vi "PalmSense Configure EIS.vi"(8 "error in (no error)":errorcluster, 10 "Message Data":variant, 11 "Data Cluster in":T1) -> (0 "error out":errorcluster, 3 "Data Cluster out":T1)   [LabVIEW 2020, in "PalmSens.lvlib"]
uses:
  PalmSens.lvlib
  PalmSense Hardware Configuration.ctl
  <instrlib>/PalmSens SDK for LabVIEW 5.10/PalmSens/PalmSens.lvclass
  support/Message Queue/Message Cluster.ctl
  support/HW Message Cluster.ctl
  C:/Program Files (x86)/National Instruments/LabVIEW 2020/instr.lib/PalmSens SDK for LabVIEW 5.10/PalmSens/Libraries/PalmSens.Core.dll
  support/Message Queue/Message Queue.lvlib
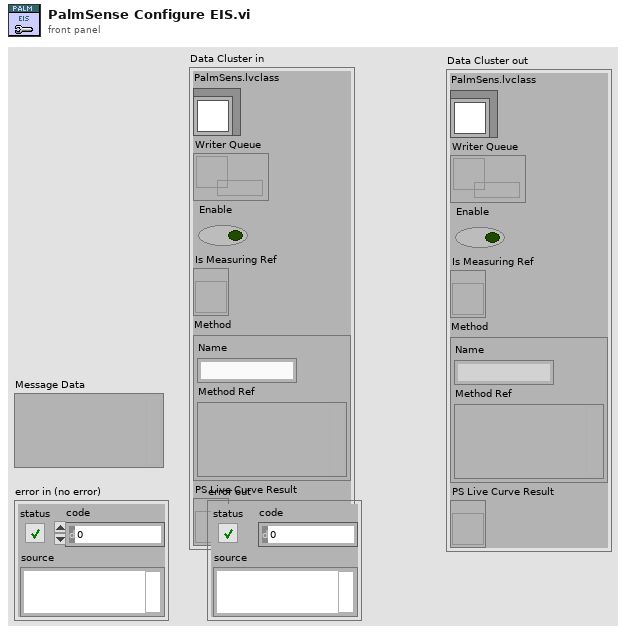
[diagram p1: front panel]
types:
  T1 = typedef "PalmSens.lvlib/PalmSense Hardware Configuration.ctl" = cluster{"PalmSens.lvclass":refnum<class "PalmSens.lvclass">, "Writer Queue":refnum<queue>, "Enable":bool, "Is Measuring Ref":refnum<vi>, "Method":cluster{"Name":string, "Method Ref":variant}, "PS Live Curve Result":refnum<vi>}
  T2 = typedef "Message Queue.lvlib/HW Message Cluster.ctl" = cluster{"Writer Queue":refnum<queue>, "Writer Data":T3}
  T3 = typedef "Message Queue.lvlib/Message Cluster.ctl" = cluster{"Message":string, "Message Data":variant}
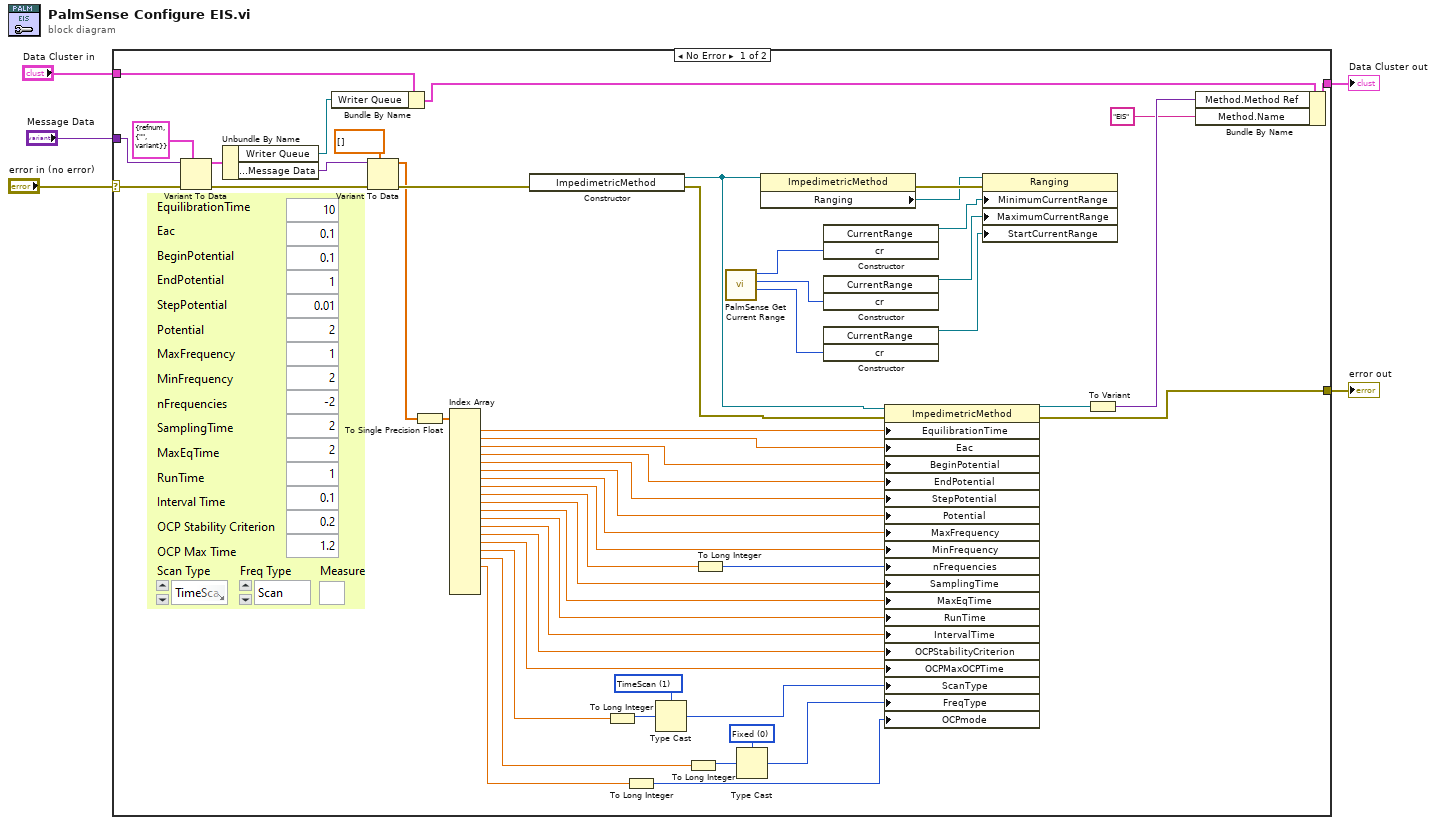
[diagram p0: block diagram]
diagram:
  n1 = case shown="No Error" "error in (no error)" {
    selector: "error in (no error)" -> [w56 w60]
    tunnel: "Message Data" -> [w54 _]
    tunnel: [w42 w61] -> w4
    tunnel: "Data Cluster in" -> [w58 w61]
    tunnel: [w45 w60] -> w2
    frame No Error {
      w32 = 0 items=["Fixed", "Scan"] ("FreqType")
      w34 = 1 items=["PGScan", "TimeScan", "Fixed"] ("ScanType")
      n2 = Variant To Data(error in=w56, type=T2 {"Writer Queue"=refnum, "Writer Data"={"Message"="", "Message Data"=variant}}, Variant=w54) -> (data=w57:T2, error out=w55:errorcluster)
      n3 = Unbundle By Name(w57) -> ("Writer Queue"=w52:refnum<queue>, "Writer Data.Message Data"=w53:variant)
      n4 = Bundle By Name(cluster=w58, "Writer Queue"=w52) -> (w59:T1)
      n5 = Variant To Data(error in=w55, type=dbl[] [] ("LSV Scan"), Variant=w53) -> (data=w37:dbl[], error out=w50:errorcluster)
      n6 = To Single Precision Float(number=w37) -> (single precision float=w27:sgl[])
      n7 = Index Array(array=w27) -> (element #1=w28:sgl, element #2=w26:sgl, element #3=w25:sgl, element #4=w24:sgl, element #5=w23:sgl, element #6=w22:sgl, element #7=w21:sgl, element #8=w20:sgl, element #9=w19:sgl, element #10=w17:sgl, element #11=w16:sgl, element #12=w15:sgl, element #13=w14:sgl, element #14=w13:sgl, element #15=w12:sgl, element #16=w10:sgl, element #17=w8:sgl, element #18=w7:sgl)  [unwired: 21 in, 3 out]
      n8 = constructor class="ImpedimetricMethod"(error in=w50) -> (reference out=w48:refnum<k24>, error out=w49:errorcluster)  [unwired: 2 in, 1 out]
      n9 = To Long Integer(number=w10) -> (32bit integer=w35:i32)
      n10 = To Long Integer(number=w7) -> (32bit integer=w6:i32)
      n11 = Type Cast(type=w34, x=w35) -> (*(type *) &x=w11:i32)
      n12 = To Long Integer(number=w8) -> (32bit integer=w33:i32)
      n13 = To Long Integer(number=w19) -> (32bit integer=w18:i32)
      n14 = call "PalmSense Get Current Range.vi"() -> ("Start Current Range"=w29:i32, "Max Current Range"=w30:i32, "Min Current Range"=w31:i32)  [unwired: 9 in]
      n15 = Type Cast(type=w32, x=w33) -> (*(type *) &x=w9:i32)
      n16 = property class="ImpedimetricMethod"(reference=w48) -> (error out=w47:errorcluster, "Ranging"=w46:refnum<k24>)  [unwired: 1 in, 1 out]
      n17 = constructor class="CurrentRange"("cr"=w31) -> (reference out=w36:refnum<k24>)  [unwired: 3 in, 3 out]
      n18 = constructor class="CurrentRange"("cr"=w30) -> (reference out=w44:refnum<k24>)  [unwired: 3 in, 3 out]
      n19 = constructor class="CurrentRange"("cr"=w29) -> (reference out=w43:refnum<k24>)  [unwired: 3 in, 3 out]
      n20 = property class="ImpedimetricMethod"(reference=w48, error in=w49, "EquilibrationTime"=w28, "Eac"=w26, "BeginPotential"=w25, "EndPotential"=w24, "StepPotential"=w23, "Potential"=w22, "MaxFrequency"=w21, "MinFrequency"=w20, "nFrequencies"=w18, "SamplingTime"=w17, "MaxEqTime"=w16, "RunTime"=w15, "IntervalTime"=w14, "OCPStabilityCriterion"=w13, "OCPMaxOCPTime"=w12, "ScanType"=w11, "FreqType"=w9, "OCPmode"=w6) -> (reference out=w41:refnum<k24>, error out=w45:errorcluster)
      n21 = property class="Ranging"(reference=w46, error in=w47, "MinimumCurrentRange"=w36, "MaximumCurrentRange"=w44, "StartCurrentRange"=w43) -> ()  [unwired: 2 out]
      n22 = To Variant(anything=w41) -> (Variant=w40:variant)
      n23 = Bundle By Name(cluster=w59, "Method.Method Ref"=w40, "Method.Name"="EIS") -> (w42:T1)
    }
    frame Error {
    }
  }
  "Data Cluster out" <- w4
  "error out" <- w2
